vi "DAQmx WAV File on AO Channel.vi"() -> ()   [LabVIEW 2011]
uses:
  <vilib>/sound/lvsound.llb/Sound Format.ctl
  <vilib>/Utility/error.llb/DialogType.ctl
  <vilib>/DAQmx/write.llb/DAQmx Write (Analog 1D DBL 1Chan NSamp).vi
  <vilib>/DAQmx/create/channels.llb/DAQmx Create Channel (AO-Voltage-Basic).vi
  <vilib>/DAQmx/configure/timing.llb/DAQmx Timing (Sample Clock).vi
  <vilib>/DAQmx/miscellaneous.llb/DAQmx Fill In Error Info.vi
panel:
  out "sound format":T1
  in  "Update Rate":dbl=8000.0 format="%0.2f"
  in  "wave file path":path=path "Select Wav File"
  in  "stop":bool
  in  "Minimum Value":dbl=-1.0 format="%0.2f"
  in  "Maximum Value":dbl=2.0 format="%0.2f"
  in  "Physical Channel":tag="Dev1/ao0"
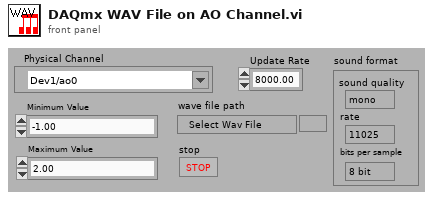
[diagram p1: front panel]
types:
  T1 = typedef "Sound Format.ctl" = cluster{"sound quality":enum16{"mono", "stereo"}, "rate":enum16{"11025", "22050", "44100", "8000"}, "bits per sample":enum16{"8 bit", "16 bit"}}
  T2 = typedef "DialogType.ctl" = u16
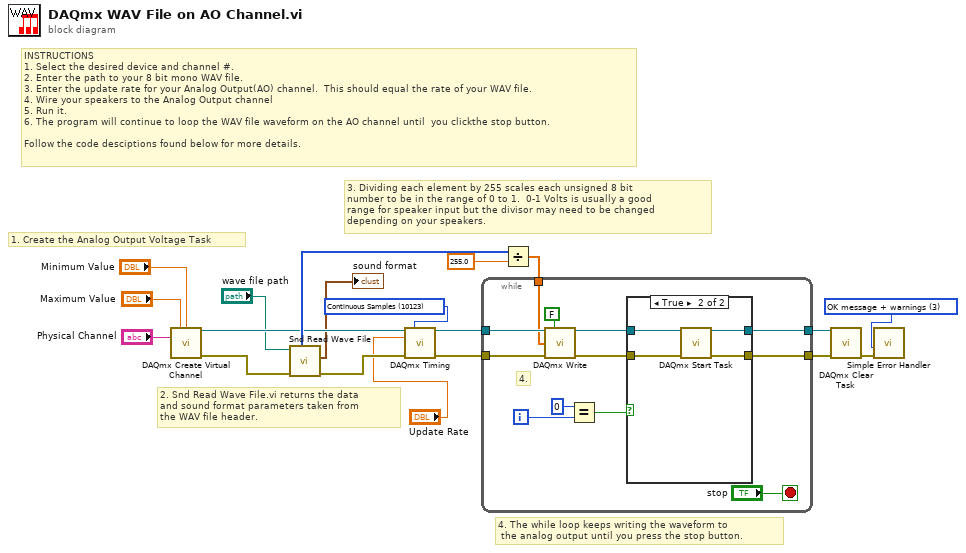
[diagram p0: block diagram]
diagram:
  w8 = 10123 items=["Finite Samples"=10178, "Continuous Samples"=10123] ("sample mode")
  w14 = T2 3 items=["no dialog", "OK message", "continue or stop message", "OK message + warnings", "continue/stop + warnings"] ("type of dialog (OK msg:1)")
  # "4. The while loop keeps writing the waveform to\n the analog output until you press the stop button."
  # "1. Create the Analog Output Voltage Task"
  # "2. Snd Read Wave File.vi returns the data\nand sound format parameters taken from \nthe WAV file header."
  # "3. Dividing each element by 255 scales each unsigned 8 bit\nnumber to be in the range of 0 to 1.  0-1 Volts is usually a good\nrange for speaker input but the divisor may need to be changed \ndepending on your speakers."
  # "INSTRUCTIONS\n1. Select the desired device and channel #.\n2. Enter the path to your 8 bit mono WAV file. \n3. Enter the update rate for your Analog Output(AO) channel.  This should equal the rate of your WAV file.\n4. Wire your speakers to the Analog Output channel \n5. Run it.\n6. The program will continue to loop the WAV file waveform on the AO channel until  you clickthe stop button.\n\nFollow the code desciptions found below for more details."
  n1 = call-poly <vilib>:"DAQmx Create Virtual Channel.vi"("maximum value"="Maximum Value", "minimum value"="Minimum Value", "physical channels"="Physical Channel") -> ("task out"=w11:refnum<k21>, "error out"=w7:errorcluster)  [unwired: 11 in]
  n2 = call <vilib>:"Snd Read Wave File.vi"("error in (no error)"=w7, "wave file path"="wave file path") -> ("error out"=w19:errorcluster, "sound format"=→"sound format":T1, "mono 8-bit"=w17:u8[])  [unwired: 3 in, 4 out]
  n3 = call-poly <vilib>:"DAQmx Timing.vi"("task/channels in"=w11, "sample mode"=w8, "rate"="Update Rate", "error in"=w19) -> ("task out"=w10:refnum<k21>, "error out"=w9:errorcluster)  [unwired: 10 in]
  n4 = Divide(x=w17, y=255.0) -> (x/y=w6:dbl[])
  n5 = while {
    tunnel: w10 -> [w30]
    tunnel: w9 -> [w29]
    tunnel: w6 -> [w27]
    tunnel: [w20] -> w5
    tunnel: [w21] -> w4
    i -> [w24]
    stop <- "stop" stop-if-true
    # "4."
    n6 = call-poly <vilib>:"DAQmx Write.vi"("task/channels in"=w30, "auto start"=FALSE, "data"=w27, "error in"=w29) -> ("task out"=w26:refnum<k21>, "error out"=w25:errorcluster)  [unwired: 9 in, 1 out]
    n7 = Equal?(x=0, y=w24) -> (x = y?=w22:bool)
    n8 = case shown="True" w22 {
      tunnel: w26 -> [w32 w37]
      tunnel: w25 -> [w33 w36]
      tunnel: [w33 w35] -> w21
      tunnel: [w32 w34] -> w20
      frame False {
      }
      frame True {
        n9 = call <vilib>:"DAQmx Start Task.vi"("task/channels in"=w37, "error in"=w36) -> ("task out"=w34:refnum<k21>, "error out"=w35:errorcluster)  [unwired: 12 in]
      }
    }
  }
  n10 = call <vilib>:"DAQmx Clear Task.vi"("task in"=w5, "error in"=w4) -> ("error out"=w15:errorcluster)  [unwired: 13 in]
  n11 = call <vilib>:"Simple Error Handler.vi"("type of dialog (OK msg:1)"=w14, "error in (no error)"=w15) -> ()  [unwired: 3 in, 5 out]
